vi "RT Main.vi"() -> ()   [LabVIEW 2021]
doc: "Demonstrates the use of the Network Streams functions to receive LED status from the host computer."
uses:
  <vilib>/myRIO/Express VI/Onboard Devices/LED/LED Express VI.xnode
  <vilib>/ErrorRing/Error Ring.xnode
  <vilib>/myRIO/Instrument Drivers/Onboard IO/DIO/vis/Write.vi
  <vilib>/myRIO/Instrument Drivers/Onboard IO/DIO/DIO.lvlib
  <vilib>/myRIO/Common/Instrument Driver Framework/myRIO v1.0/DIO/typedefs/DIO Channels Enum.ctl
  <vilib>/myRIO/Common/Instrument Driver Framework/myRIO v1.0/DIO/typedefs/DIO Channels List.ctl
  <vilib>/myRIO/Common/Instrument Driver Framework/Utilities/typedefs/Generic FPGA Reference.ctl
  <vilib>/myRIO/Common/Instrument Driver Framework/Utilities/typedefs/myRIO v1.0 Reference.ctl
  <vilib>/myRIO/Common/Instrument Driver Framework/Utilities/typedefs/Hardware Version Enum.ctl
  <vilib>/myRIO/Common/Instrument Driver Framework/Utilities/typedefs/myRIO Generic Hardware Reference.ctl
  <vilib>/myRIO/Instrument Drivers/Onboard IO/DIO/typedefs/DIO Reference.ctl
  <vilib>/myRIO/Instrument Drivers/Onboard IO/DIO/vis/myRIO DIO Open.xnode
  <vilib>/myRIO/Common/Instrument Driver Framework/Utilities/vis/Is FPGA Ref Available.vi
  <vilib>/myRIO/Instrument Drivers/Utilities/Utilities.lvlib
  <vilib>/myRIO/Common/Instrument Driver Framework/myRIO v1.0/DIO/vis/myRIO v1.2 Open DIO.vi
  <vilib>/userdefined/High Color/nirio_resource_hc.ctl
panel:
  out "LED Status":bool[](array[boolean])
  out "error out":errorcluster
  in  "Stop":bool
  # "Overview: Demonstrates the use of the Network Streams functions to receive LED status from the host computer.\nInstructions:\n1. Ensure Desktop Main.vi is already running.\n2. Run this VI.\n3. Observe the LEDs on the myRIO and the value of LED Status on this VI. They change when the value of Tank on the Desktop Main.vi changes.\n4. Click Stop to stop this VI. Stopping this VI also terminates the running of Desktop Main.vi."
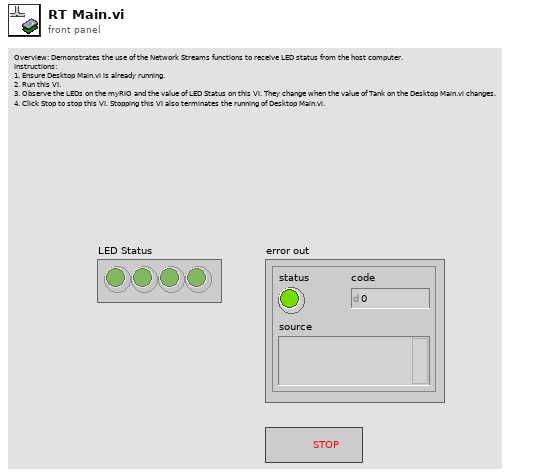
[diagram p1: front panel]
types:
  T1 = typedef "DIO.lvlib/DIO Reference.ctl" = cluster{"myRIO Reference":T2, "DIO Channels List":T6}
  T2 = typedef "myRIO Generic Hardware Reference.ctl" = cluster{"myRIO Model":T3, "myRIO Hardware Reference":T4}
  T3 = typedef "Hardware Version Enum.ctl" = enum16{"Unknown", "myRIO-1900", "myRIO-1950", "roboRIO", "NI ELVIS RIO CM", "ELVIS III"}
  T4 = typedef "myRIO v1.0 Reference.ctl" = cluster{"Generic FPGA Reference":T5, "Allow multiple opens":bool}
  T5 = typedef "Generic FPGA Reference.ctl" = refnum<k20>
  T6 = typedef "DIO Channels List.ctl" = T7[]
  T7 = typedef "DIO Channels Enum.ctl" = enum16{"Not Connected", "C/DIO0", "C/DIO1", "C/DIO2", "C/DIO3", "C/DIO4", "C/DIO5", "C/DIO6", "C/DIO7", "A/DIO0", "A/DIO1", "A/DIO2", "A/DIO3", "A/DIO4", "A/DIO5", "A/DIO6", "A/DIO7", "A/DIO8", "A/DIO9", "A/DIO10", "A/DIO11", "A/DIO12", "A/DIO13", "A/DIO14", "A/DIO15", "A/DIO16", "A/DIO17", "A/DIO18", "A/DIO19", "B/DIO0", "B/DIO1", "B/DIO2", "B/DIO3", "B/DIO4", "B/DIO5", "B/DIO6", "B/DIO7", "B/DIO8", "B/DIO9", "B/DIO10", "B/DIO11", "B/DIO12", "B/DIO13", "B/DIO14", "B/DIO15", "B/DIO16", "B/DIO17", "B/DIO18", "B/DIO19", "LED0", "LED1", "LED2", "LED3", "Button0", "DIO/DIO0", "DIO/DIO1", "DIO/DIO2", "DIO/DIO3", "DIO/DIO4", "DIO/DIO5", "DIO/DIO6", "DIO/DIO7", "DIO/DIO8", "DIO/DIO9", "SPI/CS0", "SPI/CS1", "SPI/CS2", "SPI/CS3", "LED RADIO (Green)", "LED RADIO (Red)", "LED COMM (Green)", "LED COMM (Red)", "LED MODE (Green)", "LED MODE (Red)"}
  T8 = typedef "nirio_resource_hc.ctl" = tag
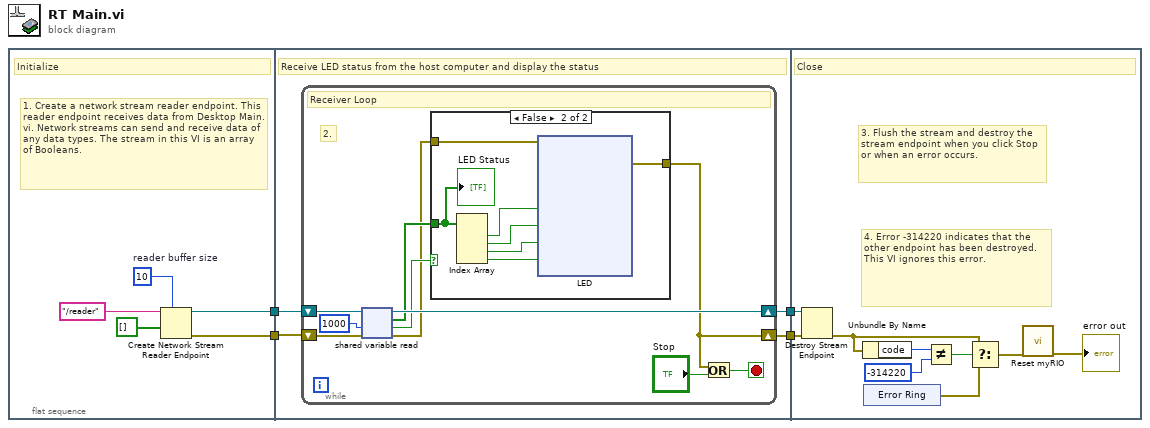
[diagram p0: block diagram]
diagram:
  n1 = flat-sequence {
    tunnel: [w7] -> w3
    tunnel: [w6] -> w2
    tunnel: [w10] -> w4
    tunnel: w3 -> [w13]
    tunnel: w2 -> [w12]
    tunnel: [w11] -> w1
    tunnel: w4 -> [w78]
    tunnel: w1 -> [w77]
    frame #0 {
      w9 = 10  # reader buffer size
      # "1. Create a network stream reader endpoint. This reader endpoint receives data from Desktop Main.vi. Network streams can send and receive data of any data types. The stream in this VI is an array of Booleans."
      # "Initialize"
      n2 = Create Network Stream Reader Endpoint(7:w9, 9:bool[] [], 11:"/reader" ("reader name")) -> (0:w6:errorcluster, 3:w7:refnum<k21>)  [unwired: 4 in]
    }
    frame #1 {
      # "Receive LED status from the host computer and display the status"
      n3 = while {
        shift-right: [w23] -> w10
        shift-left: w13 -> [w17]
        shift-right: [w14] -> w11
        shift-left: w12 -> [w20]
        stop <- w21 stop-if-true
        # "2."
        # "Receiver Loop"
        n4 = shared-variable-read(w17, w20, 1000 ("timeout ms (-1)")) -> (w23:refnum<k21>, w15:errorcluster, w16:bool, w18:bool[])
        n5 = case shown="False" w16 {
          tunnel: w18 -> [_ w30]
          tunnel: w15 -> [w24 w26]
          tunnel: [w24 w25] -> w14
          frame True {
            # "time out occurs, no data is received"
          }
          frame False {
            n6 = Index Array(array=w30) -> (element #1=w31:bool, element #2=w29:bool, element #3=w28:bool, element #4=w27:bool)  [unwired: 4 in]
            n7 = xnode "LED"("LED0"=w31, "LED1"=w29, "LED2"=w28, "LED3"=w27, "error in (no error)"=w26) -> ("error out"=w25:errorcluster)
            "LED Status" <- w30
          }
        }
        n8 = Or(x=w14, y="Stop") -> (x .or. y?=w21:bool)
      }
    }
    frame #2 {
      # "4. Error -314220 indicates that the other endpoint has been destroyed. This VI ignores this error."
      # "3. Flush the stream and destroy the stream endpoint when you click Stop or when an error occurs."
      # "Close"
      n9 = Destroy Stream Endpoint(8:w77, 11:w78) -> (0:w72:errorcluster)
      n10 = Unbundle By Name(w72) -> ("code"=w76:i32)
      n11 = xnode "Error Ring"() -> ("error out"=w73:errorcluster)
      n12 = Not Equal?(x=w76, y=-314220) -> (x != y?=w74:bool)
      n13 = Select(t=w72, s=w74, f=w73) -> (s? t:f=w71:errorcluster)
      n14 = call <vilib>:"Reset myRIO.vi"("error in (no error)"=w71) -> ("error out"=→"error out":errorcluster)  [unwired: 10 in]
    }
  }
